vi "5.2.vi"() -> ()   [LabVIEW 2023]
panel:
  in  "stop":bool
  in  "stop (T)":bool=TRUE
  out "Waveform Graph 2":dynamicdata(graph)
  out "Waveform Graph 1":dynamicdata(graph)
  in  "Forward":bool
  in  "Backward":bool
  in  "Duty Cycle (%)":dbl=50.0
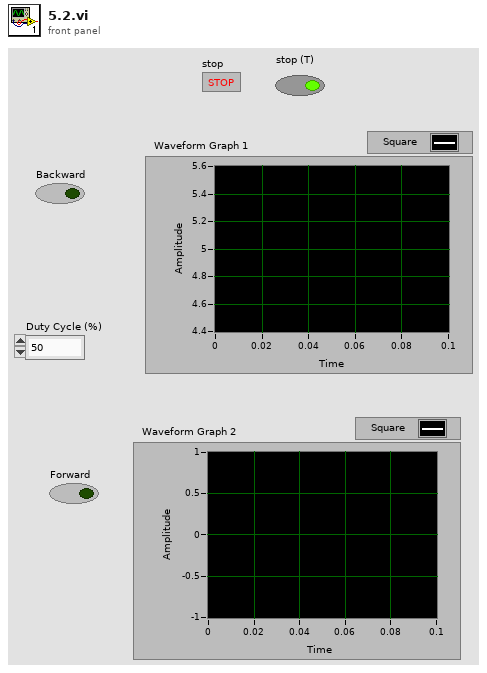
[diagram p1: front panel]
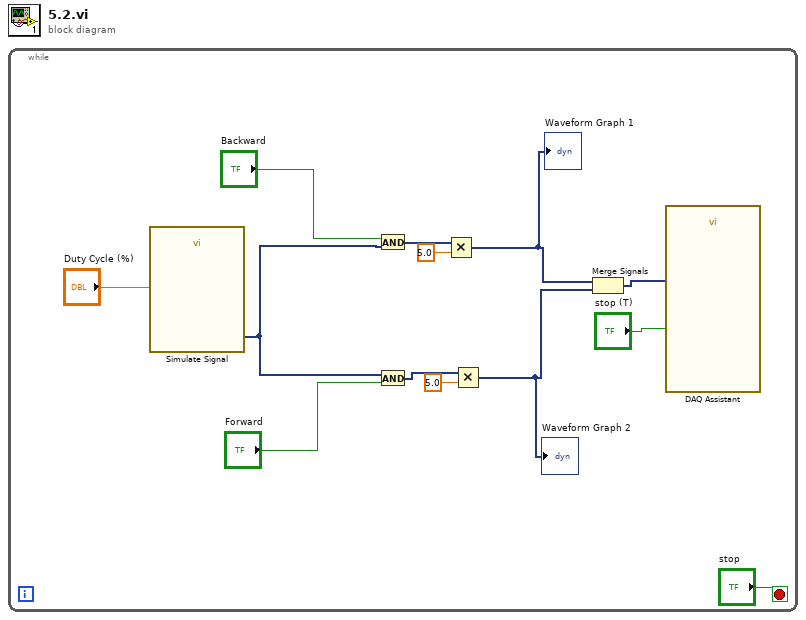
[diagram p0: block diagram]
diagram:
  n1 = while {
    stop <- "stop" stop-if-true
    n2 = call "Simulate Signal"("Duty Cycle (%)"="Duty Cycle (%)") -> ("Square"=w11:dynamicdata)  [unwired: 13 in, 1 out]
    n3 = And(x="Backward", y=w11) -> (x .and. y?=w9:dynamicdata)
    n4 = And(x=w11, y="Forward") -> (x .and. y?=w7:dynamicdata)
    n5 = Multiply(x=w9, y=5.0) -> (x*y=w4:dynamicdata)
    "Waveform Graph 1" <- w4
    n6 = Multiply(x=w7, y=5.0) -> (x*y=w3:dynamicdata)
    "Waveform Graph 2" <- w3
    n7 = Merge Signals(w4, w3) -> (w2:dynamicdata)
    n8 = call "DAQ Assistant"("data"=w2, "stop (T)"="stop (T)") -> ()  [unwired: 16 in, 2 out]
  }
